vi "Get Sciscan Scope Image Averaging.vi"(8 "error in":errorcluster, 11 "GFG Refnum":refnum<vi>) -> (0 "error out":errorcluster, 1 "Frames":i8, 2 "Type":u16(ring) items=["No Average", "Group Average", "Moving Average"], 3 "GFG Refnum Out":refnum<vi>)   [LabVIEW 2012, in "Sciscan Scope Daemon.lvlib"]
uses:
  Sciscan Scope Daemon.lvlib
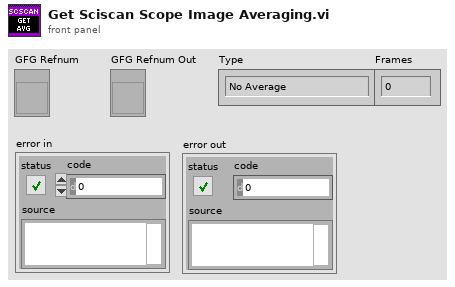
[diagram p1: front panel]
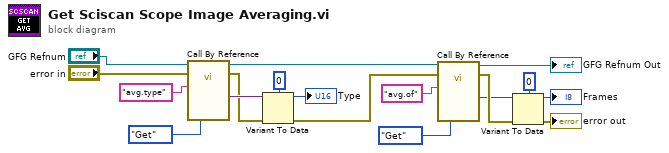
[diagram p0: block diagram]
diagram:
  n1 = call-by-ref "?"(reference="GFG Refnum", error in="error in", "Variable Name in"="avg.type", "Action"=enum16{"Init", "Set", "Get"}."Get") -> (reference out=w6:refnum<vi>, error out=w7:errorcluster, "Variant Out"=w9:variant)  [unwired: 11 in, 6 out]
  n2 = Variant To Data(error in=w7, type=u16 0 ("display every n-th frame"), Variant=w9) -> (data=→"Type":u16, error out=w5:errorcluster)
  n3 = call-by-ref "?"(reference=w6, error in=w5, "Variable Name in"="avg.of", "Action"=enum16{"Init", "Set", "Get"}."Get") -> (reference out=→"GFG Refnum Out":refnum<vi>, error out=w15:errorcluster, "Variant Out"=w14:variant)  [unwired: 11 in, 6 out]
  n4 = Variant To Data(error in=w15, type=i8 0 ("display every n-th frame"), Variant=w14) -> (data=→"Frames":i8, error out=→"error out":errorcluster)
